vi "setUp.vi"(8 "error in (no error)":errorcluster, 11 "reference in":refnum<class "Scan Engine System Tests.lvclass">) -> (0 "error out":errorcluster, 3 "reference out":refnum<class "Scan Engine System Tests.lvclass">)   [LabVIEW 2016, in "Scan Engine System Tests.lvclass"]
doc: "setUp runs prior to the test method during test execution. Use this method to initialize any object data required by your tests."
uses:
  Scan Engine System Tests.lvclass
  C:/Program Files (x86)/National Instruments/LabVIEW 2016/vi.lib/addons/_JKI Toolkits/VI Tester/TestCase.llb/TestCase.lvclass
  <vilib>/addons/_JKI Toolkits/VI Tester/TestCase.llb/TestCase.lvclass
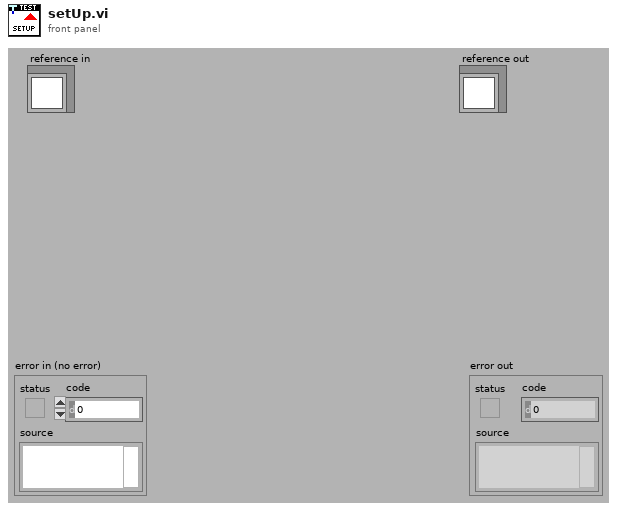
[diagram p1: front panel]
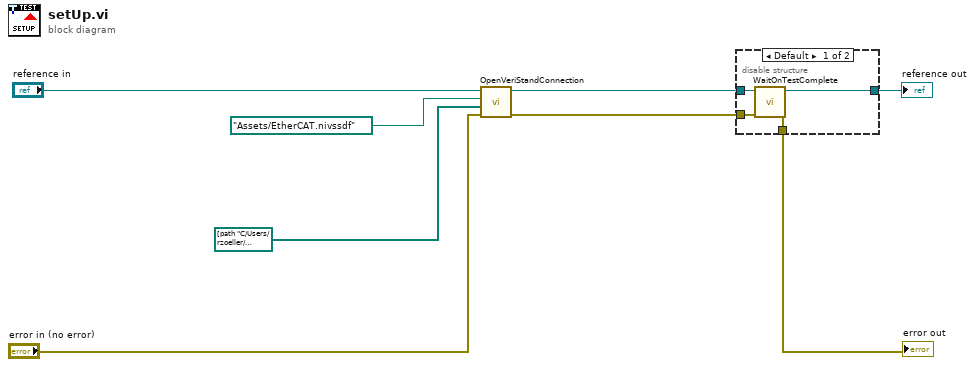
[diagram p0: block diagram]
diagram:
  n1 = call-dynamic "OpenVeriStandConnection.vi"("error in (no error)"="error in (no error)", "overrides files"=path[] [path "C:/Users/rzoeller/Documents/rzoeller-seecd/Custom Device Source/Tests/System/Assets/overrides.ini"], "System Definition File"=path "Assets/EtherCAT.nivssdf", "VeriStand Test Case in"="reference in") -> ("error out"=w3:errorcluster, "VeriStand Test Case out"=w5:refnum<class "Scan Engine System Tests.lvclass">)  [unwired: 6 in]
  n2 = disable-structure shown="Default" {
    disable-tunnel: [w12 w13] -> w8
    disable-tunnel: [w11 w14] -> w7
    disable-tunnel: w5 -> [w10 w14]
    disable-tunnel: w3 -> [w9 w13]
    frame condition #0 (active) {
      n3 = call <vilib>:"WaitOnTestComplete.vi"("error in (no error)"=w9, "TestCase in"=w10) -> ("error out"=w12:errorcluster, "TestCase out"=w11:refnum<class "Scan Engine System Tests.lvclass">)  [unwired: 8 in]
    }
    frame condition #1 {
    }
  }
  "error out" <- w8
  "reference out" <- w7
